vi "Polynomial.vi"(10 "coefficients":dbl[](array[numeric]), 11 "init value":dbl format="%#_13g") -> (3 "scaled value":dbl)   [LabVIEW 2018, in "Scale.lvlib"]
uses:
  Scale.lvlib
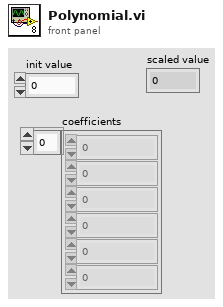
[diagram p1: front panel]
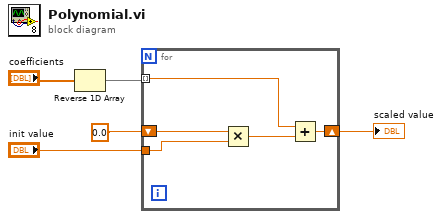
[diagram p0: block diagram]
diagram:
  n1 = Reverse 1D Array(array="coefficients") -> (reversed array=w2:dbl[])
  n2 = for {
    tunnel: w2 -> [w9] mode=indexing
    shift-right: [w8] -> w3
    shift-left: 0.0 ("double 2") -> [w7]
    tunnel: "init value" -> [w6]
    n3 = Multiply(x=w7, y=w6) -> (x*y=w10:dbl)
    n4 = Add(x=w9, y=w10) -> (x+y=w8:dbl)
  }
  "scaled value" <- w3
